vi "Send_message_to_UI.vi"(0 "Data Value Reference in":refnum<data-value>, 11 "error in (no error)":errorcluster) -> (15 "error out":errorcluster)   [LabVIEW 2019, in "Service.lvlib"]
uses:
  Service.lvlib
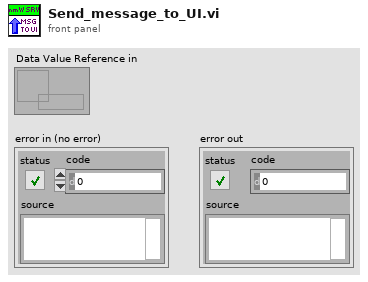
[diagram p1: front panel]
types:
  T1 = typedef "Service.lvlib/AppData.ctl" = cluster{"MsgQ":refnum<queue>, "Stop?":bool, "zmq sessions":cluster{"Control_endpoint":string, "Instr_endpoint":string}, "control-loop":cluster{"fromUI-Q":refnum<queue>, "toUI":refnum<user-event>, "Control_endpoint":string}, "UI-loop":cluster{"evnt_ref":refnum<event-registration>}, "logging":cluster{"level":dbl, "verbosity":dbl, "path":string, "Listener_ID":string}}
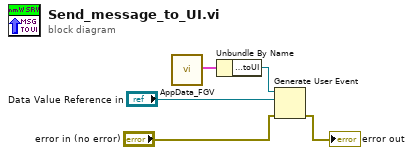
[diagram p0: block diagram]
diagram:
  n1 = call "AppData_FGV.vi"() -> ("AppData out"=w1:T1)  [unwired: 18 in, 1 out]
  n2 = Unbundle By Name(w1) -> ("control-loop.toUI"=w2:refnum<user-event>)
  n3 = Generate User Event(user event=w2, event data cluster="Data Value Reference in", error in="error in (no error)") -> (error out=→"error out":errorcluster)  [unwired: 1 in, 1 out]
